vi "Page_Advanced_WriteShared.vi"(6 "ctl references":T1, 8 "error in (no error)":errorcluster, 11 "AB_EXE in":refnum<class "AB_EXE.lvclass">) -> (0 "error out":errorcluster, 3 "AB_EXE out":refnum<class "AB_EXE.lvclass">)   [LabVIEW 2020, in "AB_EXE.lvclass"]
uses:
  <vilib>/AppBuilder/AB_Classes/EXE/AB_EXE.lvclass
  <resource>/Framework/Providers/Builds/AppBuilder/AB_UI_Page_Advanced_References.ctl
  <vilib>/AppBuilder/AB_Classes/EXE/AB_EXE.lvclass/AB_EXE.ctl
  <vilib>/AppBuilder/AB_Classes/Application/AB_Application.lvclass
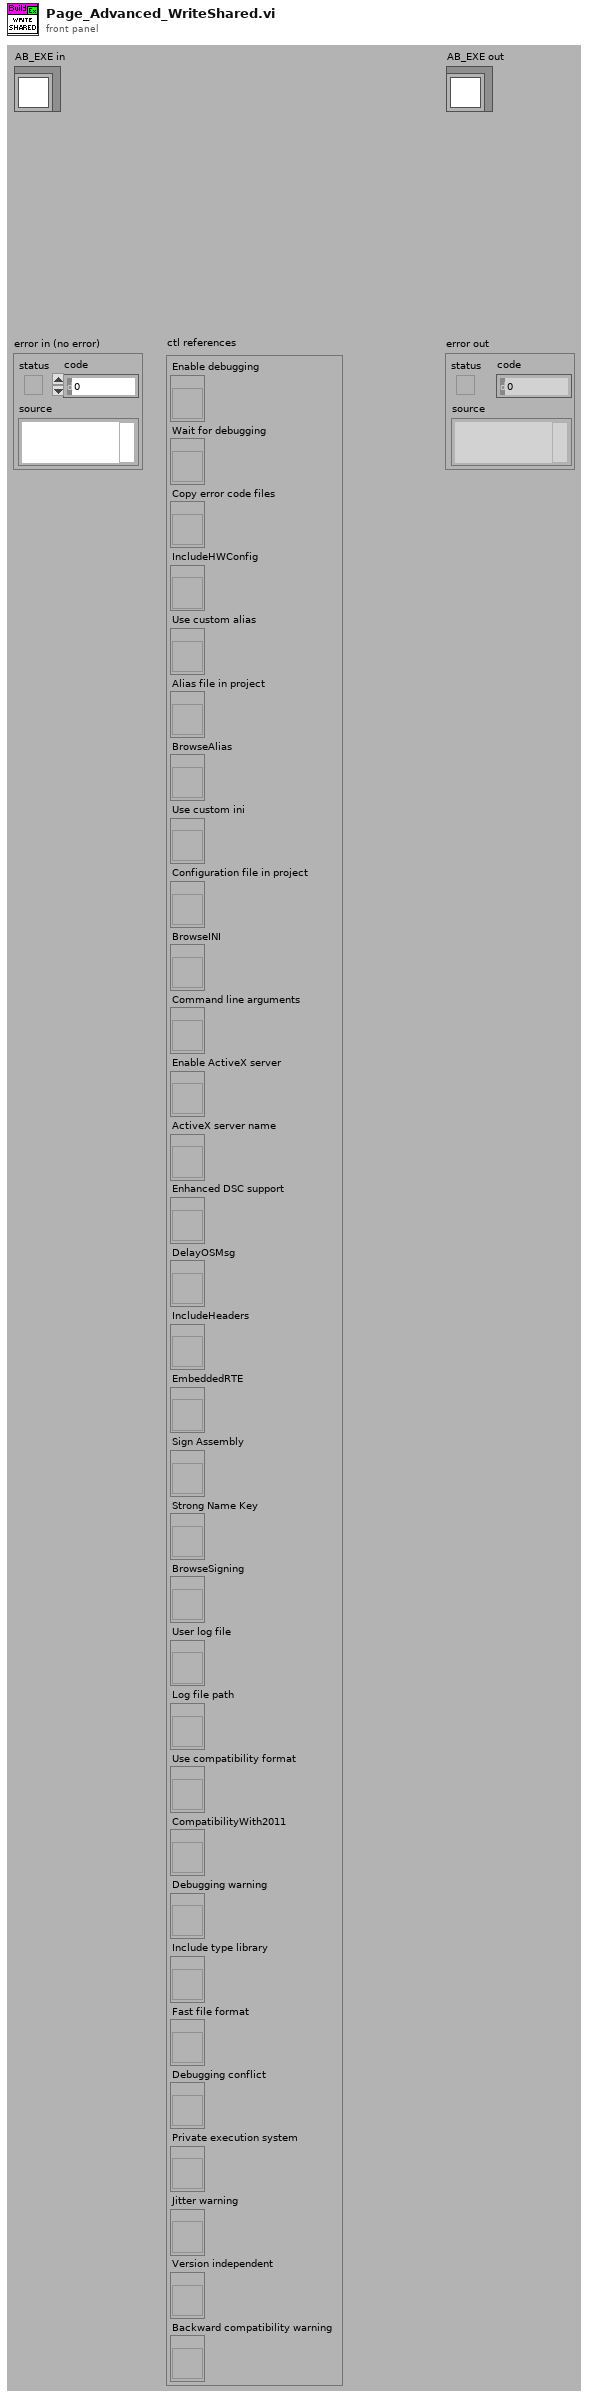
[diagram p1: front panel]
types:
  T1 = typedef "AB_UI_Page_Advanced_References.ctl" = cluster{"Enable debugging":refnum<vi>, "Wait for debugging":refnum<vi>, "Copy error code files":refnum<vi>, "IncludeHWConfig":refnum<vi>, "Use custom alias":refnum<vi>, "Alias file in project":refnum<vi>, "BrowseAlias":refnum<vi>, "Use custom ini":refnum<vi>, "Configuration file in project":refnum<vi>, "BrowseINI":refnum<vi>, "Command line arguments":refnum<vi>, "Enable ActiveX server":refnum<vi>, "ActiveX server name":refnum<vi>, "Enhanced DSC support":refnum<vi>, "DelayOSMsg":refnum<vi>, "IncludeHeaders":refnum<vi>, "EmbeddedRTE":refnum<vi>, "Sign Assembly":refnum<vi>, "Strong Name Key":refnum<vi>, "BrowseSigning":refnum<vi>, "User log file":refnum<vi>, "Log file path":refnum<vi>, "Use compatibility format":refnum<vi>, "CompatibilityWith2011":refnum<vi>, "Debugging warning":refnum<vi>, "Include type library":refnum<vi>, "Fast file format":refnum<vi>, "Debugging conflict":refnum<vi>, "Private execution system":refnum<vi>, "Jitter warning":refnum<vi>, "Version independent":refnum<vi>, "Backward compatibility warning":refnum<vi>}
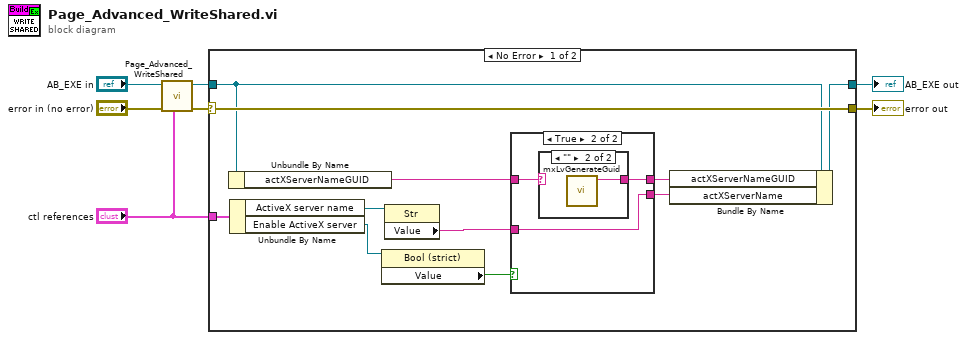
[diagram p0: block diagram]
diagram:
  n1 = call-parent "Page_Advanced_WriteShared.vi"("ctl references"="ctl references", "error in (no error)"="error in (no error)", "AB_Application in"="AB_EXE in") -> ("error out"=w4:errorcluster, "AB_Application out"=w5:refnum<class "AB_EXE.lvclass">)  [unwired: 7 out]
  n2 = case shown="No Error" w4 {
    selector: w4 -> [w18 w24]
    tunnel: w5 -> [w11 w25]
    tunnel: [w10 w25] -> w3
    tunnel: [w18 w24] -> w2
    tunnel: "ctl references" -> [w17 _]
    frame No Error {
      n3 = Unbundle By Name(w11) -> ("actXServerNameGUID"=w16:string)
      n4 = Unbundle By Name(w17) -> ("ActiveX server name"=w15:refnum<vi>, "Enable ActiveX server"=w12:refnum<vi>)
      n5 = property class="Bool (strict)"(reference=w12) -> ("Value"=w13:bool)  [unwired: 1 in, 2 out]
      n6 = property class="Str"(reference=w15) -> ("Value"=w14:string)  [unwired: 1 in, 2 out]
      n7 = case shown="True" w13 {
        tunnel: w16 -> [_ w21]
        tunnel: [_ w20] -> w9
        tunnel: w14 -> [_ w19]
        tunnel: [_ w19] -> w8
        frame False {
        }
        frame True {
          n8 = case shown="\"\"" w21 {
            selector: w21 -> [w22 _]
            tunnel: [w22 w23] -> w20
            frame Default {
            }
            frame "" {
              n9 = call <resource>:"mxLvGenerateGuid.vi"() -> ("Value"=w23:string)  [unwired: 1 in, 10 out]
            }
          }
        }
      }
      n10 = Bundle By Name(cluster=w11, "actXServerNameGUID"=w9, "actXServerName"=w8) -> (w10:refnum<class "AB_EXE.lvclass">)
    }
    frame Error {
    }
  }
  "error out" <- w2
  "AB_EXE out" <- w3
